vi "Get Test Config File.vi"(8 "error in (no error)":errorcluster, 10 "File Content":string, 11 "Configuration Manager Test in":refnum<class "Configuration Manager Test.lvclass">) -> (0 "error out":errorcluster, 2 "File Path":path, 3 "Configuration Manager Test out":refnum<class "Configuration Manager Test.lvclass">)   [LabVIEW 2020, in "Configuration Manager Test.lvclass"]
uses:
  Configuration Manager Test.lvclass
  Configuration Manager Test.lvclass/Configuration Manager Test.ctl
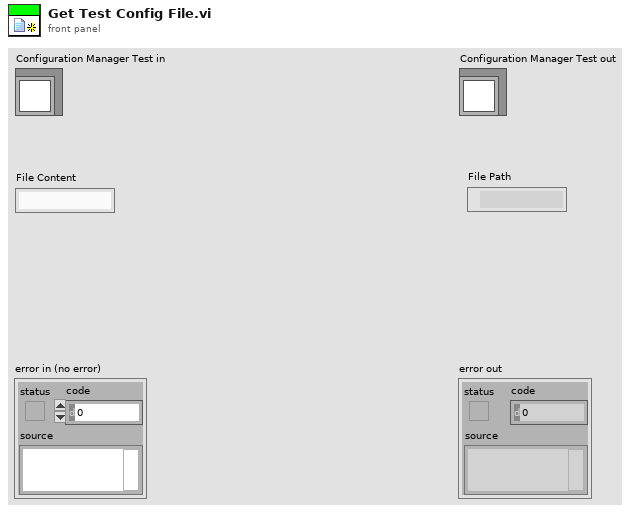
[diagram p1: front panel]
types:
  T1 = enum16{"open", "replace", "create", "open or create", "replace or create", "replace or create with confirmation"}
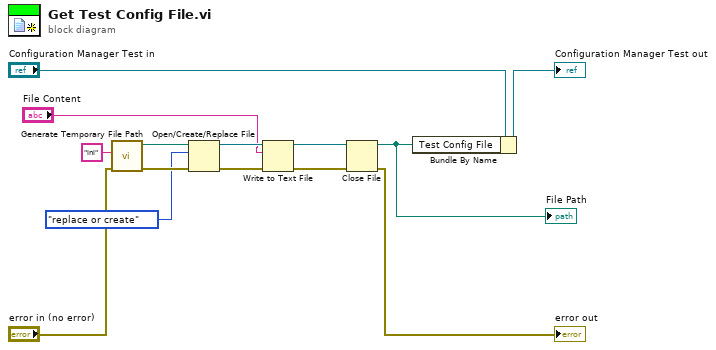
[diagram p0: block diagram]
diagram:
  n1 = call <vilib>:"Generate Temporary File Path.vi"("error in (no error)"="error in (no error)", "Temporary File Extension (tmp)"="ini") -> ("error out"=w12:errorcluster, "Unique Temporary File Path"=w13:path)  [unwired: 8 in]
  n2 = Open/Create/Replace File(file path (use dialog)=w13, error in=w12, operation (0:open)=T1."replace or create") -> (refnum out=w11:refnum<file>, error out=w10:errorcluster)  [unwired: 3 in, 1 out]
  n3 = Write to Text File(file (use dialog)=w11, text="File Content", error in=w10) -> (refnum out=w9:refnum<file>, error out=w8:errorcluster)  [unwired: 1 in, 1 out]
  n4 = Close File(refnum=w9, error in=w8) -> (path=w2:path, error out=→"error out":errorcluster)
  "File Path" <- w2
  n5 = Bundle By Name(cluster="Configuration Manager Test in", "Test Config File"=w2) -> (→"Configuration Manager Test out":refnum<class "Configuration Manager Test.lvclass">)
